vi "RemoveWindowInstance.vi"(8 "error in (no error)":errorcluster, 10 "SDL_Window *":i64, 11 "Engine in":refnum<class "Engine.lvclass">) -> (0 "error out":errorcluster, 2 "Window":refnum<class "Window.lvclass">, 3 "Engine out":refnum<class "Engine.lvclass">)   [LabVIEW 2024, in "GLF.lvlib" / "Engine.lvclass"]
uses:
  Engine.lvclass
  Window/Window.lvclass
  Engine.lvclass/Engine.ctl
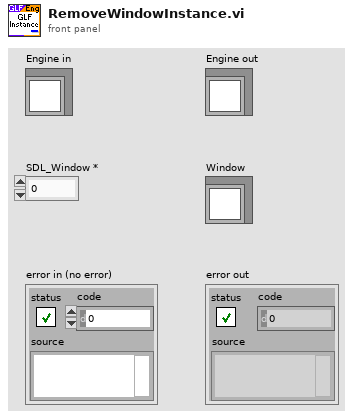
[diagram p1: front panel]
types:
  T1 = typedef "GLF.lvlib/Engine.lvclass/DVR--cluster.ctl" = cluster{"CMD Queue":T2, "Config":T3, "Ctxt":T5, "Metrics":T6, "GLF Instances":set{refnum<class "IAmGLF.lvclass">}, "Window Instances":map{i64, refnum<class "Window.lvclass">}}
  T2 = typedef "GLF.lvlib/Engine.lvclass/Command--queue.ctl" = refnum<queue>
  T3 = typedef "GLF.lvlib/Engine.lvclass/Config--cluster.ctl" = cluster{"Quit On Last Window Closed":bool, "VSync":T4, "FPS Target":dbl}
  T4 = typedef "GLF.lvlib/Engine.lvclass/VSync--enum.ctl" = enum16{"Disabled", "Enabled", "Adaptative"}
  T5 = typedef "GLF.lvlib/Engine.lvclass/Context--cluster.ctl" = cluster{"Ticks Begin":u64, "VSync Enabled":bool}
  T6 = typedef "GLF.lvlib/Engine.lvclass/Metrics--cluster.ctl" = cluster{"Uptime [ms]":u64, "Loop Time [ms]":u64}
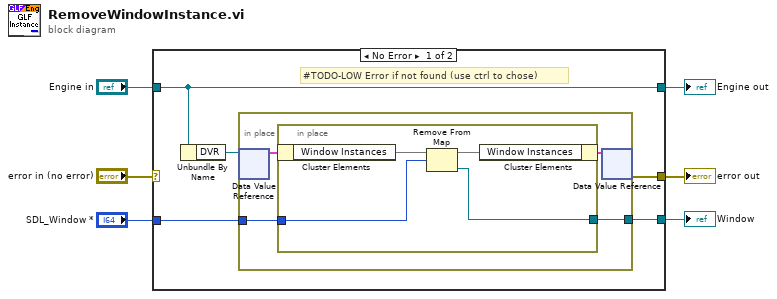
[diagram p0: block diagram]
diagram:
  n1 = case shown="No Error" "error in (no error)" {
    selector: "error in (no error)" -> [_ w21]
    tunnel: [w9 w21] -> w5
    tunnel: [w11 w20] -> w3
    tunnel: "Engine in" -> [w11 w20]
    tunnel: "SDL_Window *" -> [w8 _]
    tunnel: [w7 _] -> w1
    frame No Error {
      # "#TODO-LOW Error if not found (use ctrl to chose)"
      n2 = Unbundle By Name(w11) -> ("DVR"=w10:refnum<data-value>)
      n3 = in-place {
        in-place-border: w8 -> [w13]
        in-place-border: [w12] -> w7
        n4 = in-place-dvr #1(w10) -> (w15:T1)  [unwired: 1 out]
        n5 = in-place {
          in-place-border: w13 -> [w19]
          in-place-border: [w16] -> w12
          n6 = in-place-cluster #2(w15) -> ("Window Instances"=w18:map{i64, refnum<class "Window.lvclass">})
          n7 = Remove From Map(10:w19, 11:w18) -> (1:w16:refnum<class "Window.lvclass">, 3:w17:map{i64, refnum<class "Window.lvclass">})  [unwired: 1 out]
          n8 = in-place-cluster #2("Window Instances"=w17) -> (w14:T1)
        }
        n9 = in-place-dvr #1(w14) -> (w9:errorcluster)  [unwired: 1 out]
      }
    }
    frame Error {
    }
  }
  "error out" <- w5
  "Engine out" <- w3
  "Window" <- w1
